vi "AWS Upload (SubVI).vi"(8 "Temp Filename":string, 9 "AWS Bucket":string, 10 "Object path":string, 11 "Local File Path":string) -> (0 "error out":errorcluster, 3 "Temp Path":path)   [LabVIEW 2019]
uses:
  <vilib>/National Instruments/LabVIEW Interface for Amazon S3/LV Interface for Amazon S3.lvlib
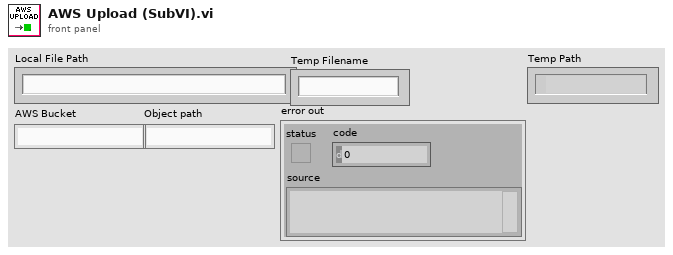
[diagram p1: front panel]
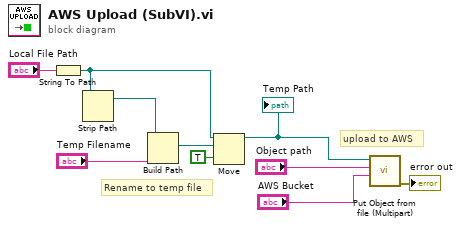
[diagram p0: block diagram]
diagram:
  # "upload to AWS"
  # "Rename to temp file"
  n1 = String To Path(string="Local File Path") -> (path=w4:path)
  n2 = Strip Path(path=w4) -> (stripped path=w8:path)  [unwired: 1 out]
  n3 = Build Path(base path=w8, name or relative path="Temp Filename") -> (appended path=w3:path)
  n4 = Move(source path=w4, 9:TRUE ("overwrite (F)"), 10:w3) -> (3:w2:path)  [unwired: 2 in, 2 out]
  "Temp Path" <- w2
  n5 = call <vilib>:"Put Object from file (Multipart).vi"("Bucket"="AWS Bucket", "Object path"="Object path", "Local file path"=w2) -> ("error out"=→"error out":errorcluster)  [unwired: 6 in, 2 out]
